vi "Calculate Statistics.vi"(8 "error in (no error)":errorcluster, 9 "Stream Names":string[](array[string]), 10 "Data":waveform(dbl)[](array[waveform]), 11 "Statistic in":refnum<class "Statistic.lvclass">) -> (0 "error out":errorcluster, 1 "Statistic Channels":string[](array[string]), 2 "Statistic Waveforms":waveform(dbl)[](array[waveform]), 3 "Statistic out":refnum<class "Statistic.lvclass">)   [LabVIEW 2025, in "Statistic.lvlib" / "Statistic.lvclass"]
uses:
  Statistic.lvclass
  Statistic.lvclass/Statistic.ctl
  <vilib>/Analysis/baseanly.llb/Mean (DBL).vi
  <vilib>/Analysis/5stat.llb/RMS (DBL).vi
  <vilib>/Analysis/NI_AALBase.lvlib
  <vilib>/Analysis/NI_AALPro.lvlib
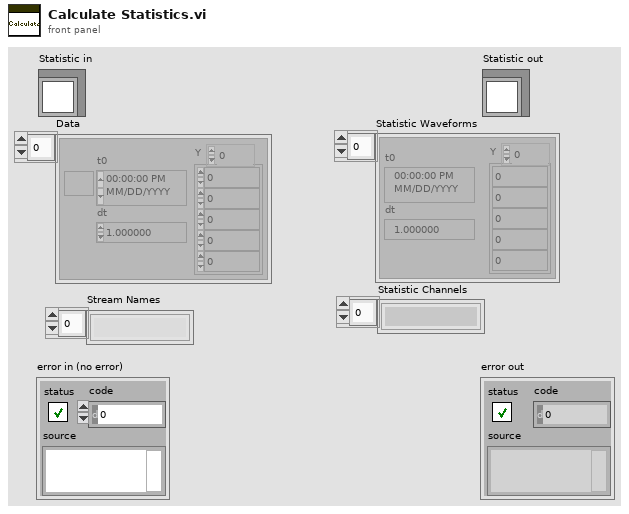
[diagram p1: front panel]
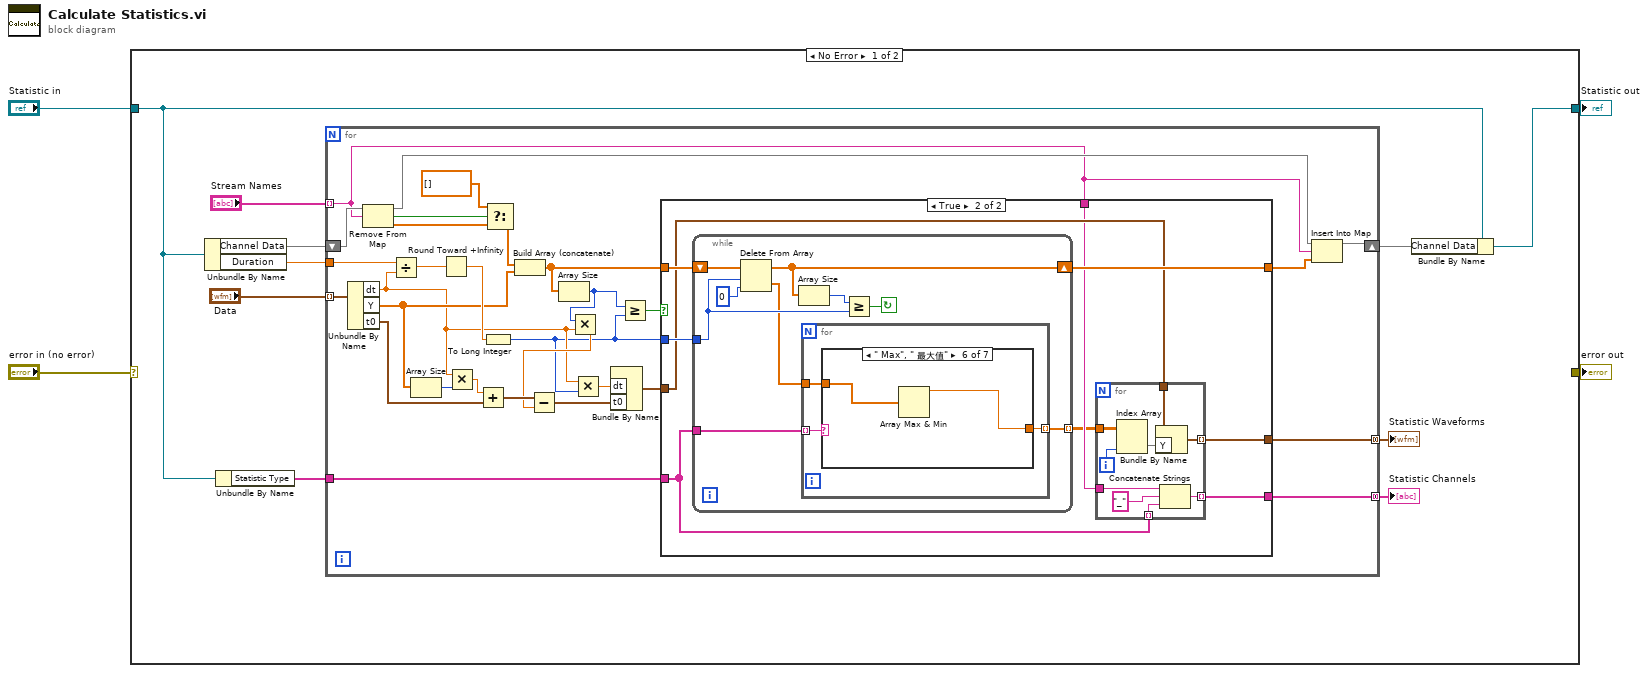
[diagram p0: block diagram]
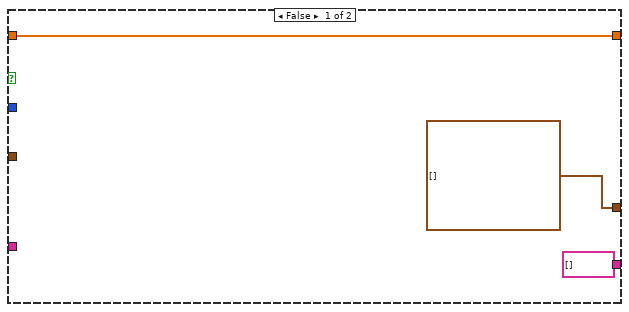
[diagram p2: hidden frame]
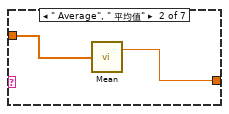
[diagram p4: hidden frame]
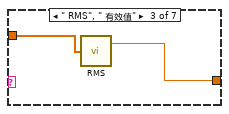
[diagram p5: hidden frame]
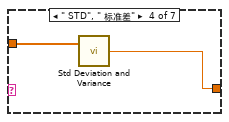
[diagram p6: hidden frame]
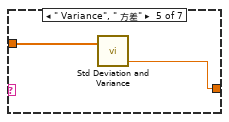
[diagram p7: hidden frame]
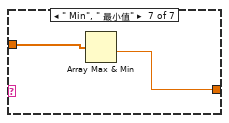
[diagram p8: hidden frame]
diagram:
  n1 = case shown="No Error" "error in (no error)" {
    selector: "error in (no error)" -> [_ w91]
    tunnel: [_ w91] -> w3
    tunnel: [w6 w90] -> w1
    tunnel: "Statistic in" -> [w5 w90]
    frame No Error {
      n2 = Unbundle By Name(w5) -> ("Channel Data"=w9:map{string, dbl[]}, "Duration"=w13:dbl)
      n3 = Unbundle By Name(w5) -> ("Statistic Type"=w7:string[])
      n4 = for {
        tunnel: "Data" -> [w44] mode=indexing
        tunnel: w13 -> [w43]
        tunnel: "Stream Names" -> [w17] mode=indexing
        tunnel: [w37] -> w11 mode=concatenating
        tunnel: [w36] -> w10 mode=concatenating
        shift-right: [w16] -> w8
        shift-left: w9 -> [w24]
        tunnel: w7 -> [w15]
        n5 = Unbundle By Name(w44) -> ("dt"=w27:dbl, "Y"=w35:dbl[], "t0"=w32:timestamp)
        n6 = Remove From Map(10:w17, 11:w24) -> (1:w21:dbl[], 2:w23:bool, 3:w19:map{string, dbl[]})
        n7 = Divide(x=w43, y=w27) -> (x/y=w42:dbl)
        n8 = Array Size(array=w35) -> (size(s)=w34:i32)
        n9 = Round Toward +Infinity(x=w42) -> (ceil(x): smallest int >= x=w39:dbl)
        n10 = Multiply(x=w27, y=w34) -> (x*y=w33:dbl)
        n11 = Add(x=w33, y=w32) -> (x+y=w31:timestamp)
        n12 = To Long Integer(number=w39) -> (32bit integer=w26:i32)
        n13 = Select(t=dbl[] [] ("array"), s=w23, f=w21) -> (s? t:f=w20:dbl[])
        n14 = Build Array (concatenate)(w20, w35) -> (w40:dbl[])
        n15 = Array Size(array=w40) -> (size(s)=w30:i32)
        n16 = Multiply(x=w30, y=w27) -> (x*y=w29:dbl)
        n17 = Subtract(x=w31, y=w29) -> (x-y=w28:timestamp)
        n18 = Multiply(x=w27, y=w26) -> (x*y=w25:dbl)
        n19 = Bundle By Name("dt"=w25, "t0"=w28) -> (w38:waveform(dbl))  [unwired: 1 in]
        n20 = Greater Or Equal?(x=w30, y=w26) -> (x >= y?=w41:bool)
        n21 = case shown="True" w41 {
          tunnel: w40 -> [w47 w56]
          tunnel: [w47 w54] -> w18
          tunnel: w26 -> [_ w55]
          tunnel: w38 -> [_ w53]
          tunnel: [waveform(dbl)[] [] w52] -> w37
          tunnel: w17 -> [_ w51]
          tunnel: [string[] [] w49] -> w36
          tunnel: w15 -> [_ w48]
          frame False {
          }
          frame True {
            n22 = while {
              shift-right: [w72] -> w54
              shift-left: w56 -> [w74]
              tunnel: w55 -> [w70]
              tunnel: [w67] -> w50 mode=indexing
              tunnel: w48 -> [w66]
              stop <- w69 continue-if-true
              n23 = Delete From Array(array=w74, length=w70, index=0) -> (deleted portion=w68:dbl[], array with subset deleted=w72:dbl[])
              n24 = Array Size(array=w72) -> (size(s)=w71:i32)
              n25 = for {
                tunnel: w68 -> [w77]
                tunnel: [w76] -> w67 mode=indexing
                tunnel: w66 -> [w75] mode=indexing
                n26 = case shown="\" Max\", \" 最大值\"" w75 {
                  tunnel: w77 -> [_ w79 w81 w83 w85 w87 w89]
                  tunnel: [_ w78 w80 w82 w84 w86 w88] -> w76
                  frame "", Default {
                  }
                  frame " Average", " 平均值" {
                    n27 = call-poly <vilib>:"Mean.vi"("X"=w79) -> ("mean"=w78:dbl)  [unwired: 1 out]
                  }
                  frame " RMS", " 有效值" {
                    n28 = call-poly <vilib>:"RMS.vi"("X"=w81) -> ("rms value"=w80:dbl)  [unwired: 1 out]
                  }
                  frame " STD", " 标准差" {
                    n29 = call <vilib>:"Std Deviation and Variance.vi"("X"=w83) -> ("standard deviation"=w82:dbl)  [unwired: 1 in, 2 out]
                  }
                  frame " Variance", " 方差" {
                    n30 = call <vilib>:"Std Deviation and Variance.vi"("X"=w85) -> ("variance"=w84:dbl)  [unwired: 1 in, 2 out]
                  }
                  frame " Max", " 最大值" {
                    n31 = Array Max & Min(array=w87) -> (max value=w86:dbl)  [unwired: 3 out]
                  }
                  frame " Min", " 最小值" {
                    n32 = Array Max & Min(array=w89) -> (min value=w88:dbl)  [unwired: 3 out]
                  }
                }
              }
              n33 = Greater Or Equal?(x=w71, y=w70) -> (x >= y?=w69:bool)
            }
            n34 = for {
              tunnel: w53 -> [w65]
              tunnel: [w64] -> w52 mode=indexing
              tunnel: w48 -> [w62] mode=indexing
              tunnel: w51 -> [w61]
              tunnel: w50 -> [w60]
              tunnel: [w57] -> w49 mode=indexing
              i -> [w59]
              n35 = Index Array(array=w60, index (col)=w59) -> (element=w58:dbl[])  [unwired: 1 in]
              n36 = Bundle By Name(cluster=w65, "Y"=w58) -> (w64:waveform(dbl))
              n37 = Concatenate Strings(w61, "_" ("string"), w62) -> (w57:string)
            }
          }
        }
        n38 = Insert Into Map(map in=w19, key=w17, value=w18) -> (map out=w16:map{string, dbl[]})  [unwired: 2 out]
      }
      "Statistic Waveforms" <- w11
      "Statistic Channels" <- w10
      n39 = Bundle By Name(cluster=w5, "Channel Data"=w8) -> (w6:refnum<class "Statistic.lvclass">)
    }
    frame Error {
    }
  }
  "error out" <- w3
  "Statistic out" <- w1
